vi "DAQ.setAmplitudeLimit.vi"(8 "error in (no error)":errorcluster, 10 "Amplitude Limit":T1 {"Limit (V)" format="%.3p"}, 11 "Instrument.DAQ":refnum<class "Instrument.DAQ.lvclass">) -> (0 "error out":errorcluster, 3 "Instrument.DAQ out":refnum<class "Instrument.DAQ.lvclass">)   [LabVIEW 2019, in "Instrument.Lockin.lvlib" / "Instrument.DAQ.lvclass"]
doc: "---------------------------------------------------------------\nJKI State Machine Objects™\nhttp://jki.net/state-machine-objects/\nCopyright (C) 2005-2015, JKI <info@jki.net>\nALL RIGHTS RESERVEDJKI State Machine Objects (SMO) 1.0.0.4\nJKI - JKI\nCopyright (c) 2015, JKI"
uses:
  Instrument.DAQ.lvclass
  Typedefs/Configuration.AmplitudeLimit--Cluster.ctl
  Instrument.DAQ.lvclass/Instrument.DAQ.ctl
  Typedefs/PrivateEvents--DAQ.setAmplitudeLimit.ctl
panel:
  # "For instructions on how to use the JKI State Machine Objects, examples and video tutorials, visit:\nhttp://jki.net/state-machine-objects/\n\nJKI State Machine Objects™\nhttp://jki.net/state-machine-objects/\nCopyright (C) 2005-2015, JKI <info@jki.net>\nALL RIGHTS RESERVED"
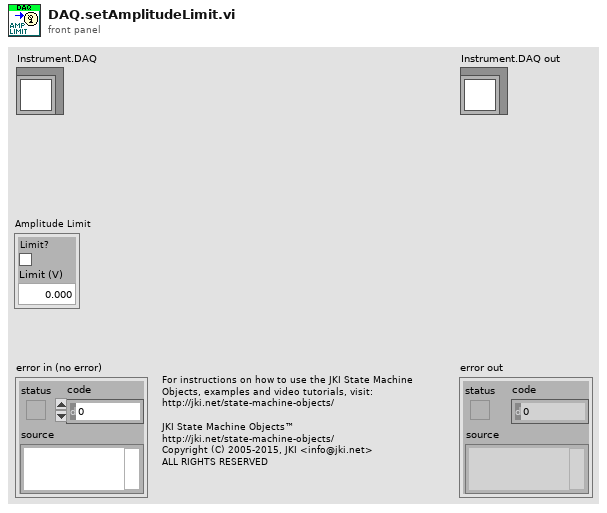
[diagram p1: front panel]
types:
  T1 = typedef "Instrument.Lockin.lvlib/Instrument.DAQ.lvclass/Configuration.AmplitudeLimit--Cluster.ctl" = cluster{"Limit?":bool, "Limit (V)":dbl}
  T2 = typedef "Instrument.Lockin.lvlib/Instrument.DAQ.lvclass/PrivateEvents--DAQ.setAmplitudeLimit.ctl" = cluster{"Amplitude Limit ":T1}
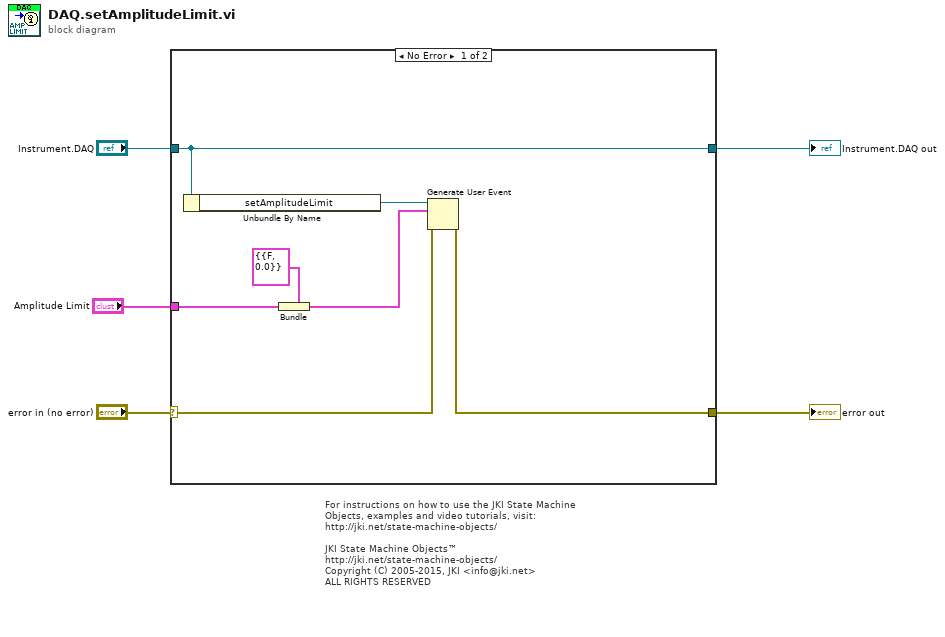
[diagram p0: block diagram]
diagram:
  # "For instructions on how to use the JKI State Machine Objects, examples and video tutorials, visit:\nhttp://jki.net/state-machine-objects/\n\nJKI State Machine Objects™\nhttp://jki.net/state-machine-objects/\nCopyright (C) 2005-2015, JKI <info@jki.net>\nALL RIGHTS RESERVED"
  n1 = case shown="No Error" "error in (no error)" {
    selector: "error in (no error)" -> [w12 w14]
    tunnel: [w10 w14] -> w4
    tunnel: [w9 w13] -> w5
    tunnel: "Instrument.DAQ" -> [w9 w13]
    tunnel: "Amplitude Limit" -> [w8 _]
    frame No Error {
      n2 = Unbundle By Name(w9) -> ("setAmplitudeLimit"=w11:refnum<user-event>)
      n3 = Bundle(cluster=T2 {"Amplitude Limit "={"Limit?"=FALSE, "Limit (V)"=0.0}} ("setAmplitudeLimit"), "Amplitude Limit"=w8) -> (w7:T2)
      n4 = Generate User Event(user event=w11, event data cluster=w7, error in=w12) -> (error out=w10:errorcluster)  [unwired: 1 in, 1 out]
    }
    frame Error {
    }
  }
  "error out" <- w4
  "Instrument.DAQ out" <- w5
